vi "LWXPS_ControllerRTTimeGet.vi"(0 "XPS Reference IN":refnum<k24>, 5 "LabVIEW error IN":errorcluster) -> (14 "XPS Reference OUT":refnum<k24>, 15 "Returned error code":i32, 16 "Current RT Period":dbl, 17 "Current RT Usage":dbl, 18 "XPS Error String":string, 19 "LabVIEW error OUT":errorcluster)   [LabVIEW 2014]
uses:
  D:/XPSQ8_LabView_Library/Development/Source/Dll/Newport.XPS.CommandInterface.dll
  Dll/Newport.XPS.CommandInterface.dll
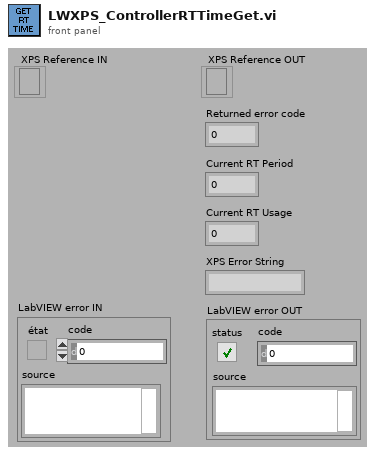
[diagram p1: front panel]
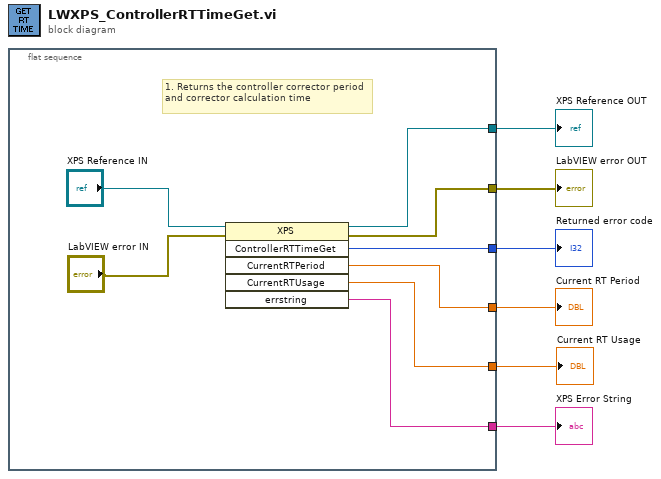
[diagram p0: block diagram]
diagram:
  n1 = flat-sequence {
    tunnel: [w7] -> w6
    tunnel: [w14] -> w5
    tunnel: [w13] -> w3
    tunnel: [w10] -> w4
    tunnel: [w9] -> w2
    tunnel: [w8] -> w1
    frame #0 {
      # "1. Returns the controller corrector period and corrector calculation time"
      n2 = invoke class="XPS" method="ControllerRTTimeGet"(reference="XPS Reference IN", error in="LabVIEW error IN") -> (reference out=w7:refnum<k24>, error out=w14:errorcluster, "ControllerRTTimeGet"=w10:i32, "CurrentRTPeriod"=w13:dbl, "CurrentRTUsage"=w9:dbl, "errstring"=w8:string)  [unwired: 4 in]
    }
  }
  "XPS Reference OUT" <- w6
  "LabVIEW error OUT" <- w5
  "Returned error code" <- w4
  "Current RT Period" <- w3
  "Current RT Usage" <- w2
  "XPS Error String" <- w1
